vi "X-.vi"(8 "Width":dbl=20.0, 9 "Length":dbl=20.0, 10 "Z":dbl, 11 "X":dbl) -> (0 "X-":dbl, 3 "(X-)^2":dbl)   [LabVIEW 2020]
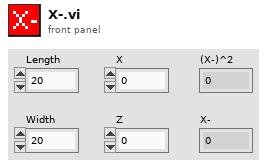
[diagram p1: front panel]
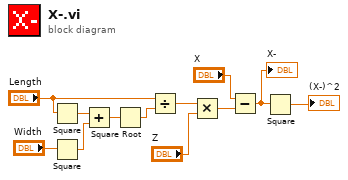
[diagram p0: block diagram]
diagram:
  n1 = Square(x="Length") -> (x^2=w4:dbl)
  n2 = Square(x="Width") -> (x^2=w3:dbl)
  n3 = Add(x=w4, y=w3) -> (x+y=w2:dbl)
  n4 = Square Root(x=w2) -> (sqrt(x)=w5:dbl)
  n5 = Divide(x="Length", y=w5) -> (x/y=w8:dbl)
  n6 = Multiply(x=w8, y="Z") -> (x*y=w10:dbl)
  n7 = Subtract(x="X", y=w10) -> (x-y=w12:dbl)
  "X-" <- w12
  n8 = Square(x=w12) -> (x^2=→"(X-)^2":dbl)
